vi "RSZVB Get Pulse Modulator.vi"(8 "error in (no error)":errorcluster {"code" format="%.0x"}, 9 "Path (1)":i32=1, 10 "Channel (1)":i32=1, 11 "VISA session":refnum<visa-resource-name>) -> (0 "error out":errorcluster {"code" format="%.0x"}, 1 "Pulse Modulator":bool, 3 "dup VISA session":refnum<visa-resource-name>)   [LabVIEW 2011]
doc: "This VI returns the state of the pulse modulators.\n\nRemote-control command(s):\n[SENSe<Ch>:]EUNit:PMODulator<Path>[:STATe]?"
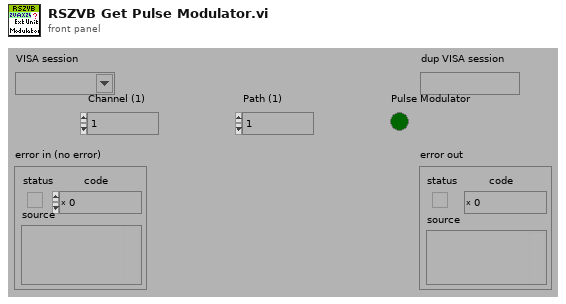
[diagram p1: front panel]
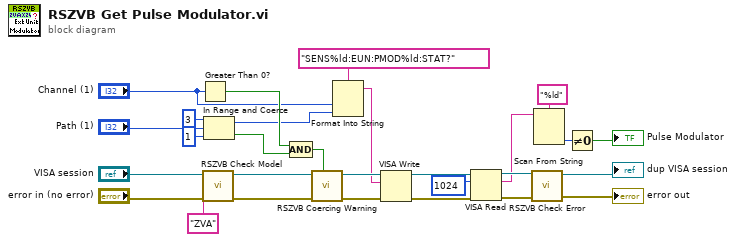
[diagram p0: block diagram]
diagram:
  n1 = Greater Than 0?(x="Channel (1)") -> (x > 0?=w19:bool)
  n2 = call "RSZVB Check Model.vi"("error in (no error)"="error in (no error)", "Model"="ZVA" ("Options"), "VISA session"="VISA session") -> ("error out"=w13:errorcluster, "dup VISA session"=w14:refnum<visa-resource-name>)  [unwired: 7 in]
  n3 = In Range and Coerce(upper limit=3, x="Path (1)", lower limit=1) -> (coerced(x)=w18:i32, In Range?=w20:bool)
  n4 = Compound Arithmetic op=AND(w19, w20) -> (w22:bool)
  n5 = call "RSZVB Coercing Warning.vi"("In Range?"=w22, "error in (no error)"=w13, "VISA session"=w14) -> ("error out"=w27:errorcluster, "dup VISA session"=w28:refnum<visa-resource-name>)  [unwired: 7 in]
  n6 = Format Into String(format string="SENS%ld:EUN:PMOD%ld:STAT?", "Channel (1)", w18) -> (resulting string=w26:string)  [unwired: 2 in, 1 out]
  n7 = VISA Write(VISA resource name=w28, write buffer=w26, error in (no error)=w27) -> (VISA resource name out=w16:refnum<visa-resource-name>, error out=w15:errorcluster)  [unwired: 1 out]
  n8 = VISA Read(VISA resource name=w16, byte count=u32 1024 ("byte count (0)"), error in (no error)=w15) -> (VISA resource name out=w12:refnum<visa-resource-name>, read buffer=w8:string, error out=w11:errorcluster)  [unwired: 1 out]
  n9 = call "RSZVB Check Error.vi"("error in (no error)"=w11, "VISA session"=w12) -> ("error out"=→"error out":errorcluster, "dup VISA session"=→"dup VISA session":refnum<visa-resource-name>)  [unwired: 8 in]
  n10 = Scan From String(format string="%ld", input string=w8) -> (output 1=w9:i32)  [unwired: 3 in, 3 out]
  n11 = Not Equal To 0?(x=w9) -> (x != 0?=→"Pulse Modulator":bool)
